vi "termometr.vi"() -> ()   [LabVIEW 2023]
uses:
  <vilib>/numeric/Random Number (Range) I64.vi
  <vilib>/numeric/sub_Random U32.vi
panel:
  in  "stop":bool
  in  "skala":bool
  out "temp. F":dbl(slide) scale=0.0..100.0 scale format="%.2g"
  out "temp. C":dbl(slide) scale=0.0..30.0 scale format="%.2g"
  # "deg C"
  # "deg F"
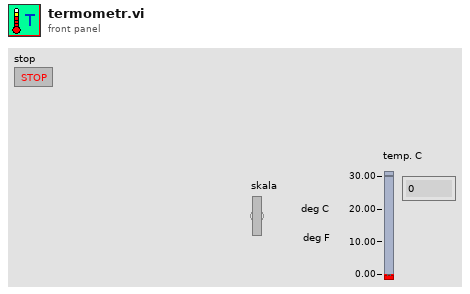
[diagram p1: front panel]
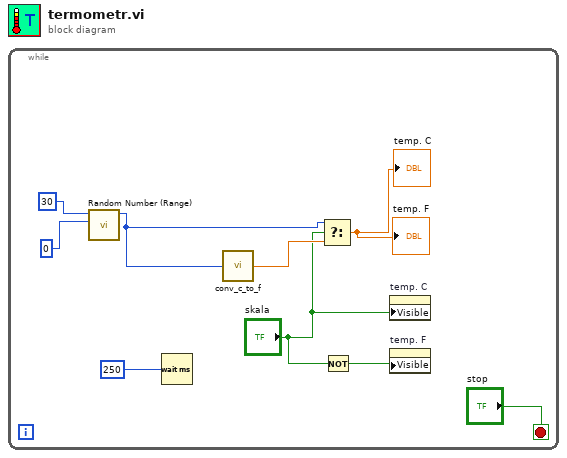
[diagram p0: block diagram]
diagram:
  n1 = while {
    stop <- "stop" stop-if-true
    n2 = call-poly <vilib>:"Random Number (Range).vi"("lower bound (-100)"=0, "upper bound (100)"=30) -> ("number"=w5:i64)  [unwired: 9 in]
    n3 = Wait (ms)(milliseconds to wait=250) -> ()  [unwired: 1 out]
    n4 = call "conv_c_to_f.vi"("deg. C"=w5) -> ("deg. F"=w7:dbl)
    n5 = Select(t=w5, s="skala", f=w7) -> (s? t:f=→"temp. C" →"temp. F":dbl)
    n6 = Not(x="skala") -> (.not. x?=w3:bool)
    n7 = property on="temp. C" class="Slide (strict)"("Visible"="skala") -> ()  [unwired: 2 in, 2 out]
    n8 = property on="temp. F" class="Slide (strict)"("Visible"=w3) -> ()  [unwired: 2 in, 2 out]
  }
